vi "Actor Core.vi"(8 "error in":errorcluster, 11 "Select Report File Dialog in":refnum<class "Select Report File Dialog.lvclass">) -> (0 "error out":errorcluster, 3 "Actor out":refnum<class "Actor.lvclass">)   [LabVIEW 2014, in "Select Report File Dialog.lvlib" / "Select Report File Dialog.lvclass"]
doc: "(<B>Filename</B>: Actor Framework.lvlib:Actor.lvclass:Actor Core.vi)\n\nReceives messages to the actor, reacts to them, and initiates any error handling that may shut the actor down.\n\nDescendant classes may override this VI to append parallel tasks for the actor to complete while it handles messages. Overrides use the Call Parent Method node."
uses:
  Select Report File Dialog.lvclass
  <vilib>/ActorFramework/Actor/Actor.lvclass
  <vilib>/ActorFramework/Actor/Actor.lvclass/Actor.ctl
  <vilib>/ActorFramework/Message Enqueuer/Message Enqueuer.lvclass/Message Enqueuer.ctl
  Select Report File Dialog Messages/Write Select Report File Msg/Write Select Report File Msg.lvclass/Write Select Report File Msg.ctl
  <vilib>/ActorFramework/Message Enqueuer/Init from Existing Queue.vi
  <vilib>/ActorFramework/Message Enqueuer/Enqueue.vi
  <vilib>/ActorFramework/Message Priority Queue/Priority Enqueue.vi
  Viewable Actor/ViewableActor/ViewableActor.lvclass
  <vilib>/ActorFramework/Message Enqueuer/Message Enqueuer.lvclass
  Select Report File Dialog Messages/Write Select Report File Msg/Write Select Report File Msg.lvclass
  <vilib>/ActorFramework/Stop Msg/Stop Msg.lvclass
panel:
  in  "Select Report File":path
  in  "Stop Signal":bool
  in  "Stop":bool
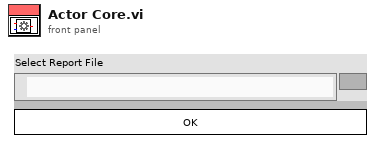
[diagram p1: front panel]
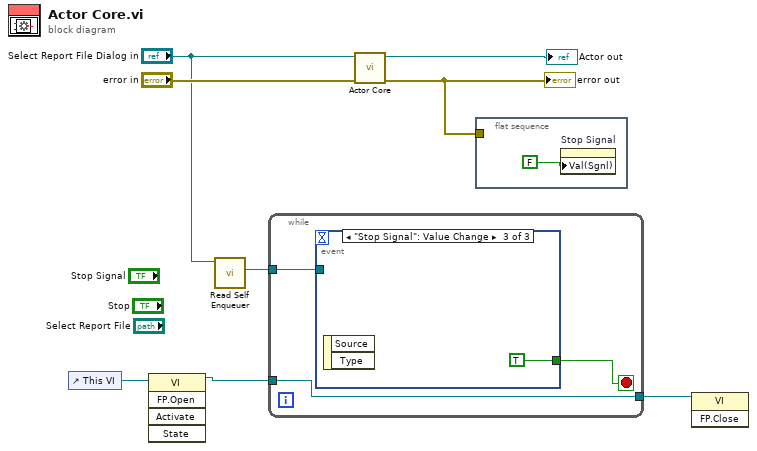
[diagram p0: block diagram]
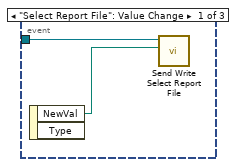
[diagram p2: hidden frame]
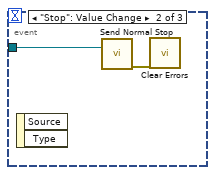
[diagram p3: hidden frame]
diagram:
  n1 = control-ref of="This VI"() -> (w3:refnum<vi>)
  n2 = invoke class="VI" method="FP.Open"(reference=w3) -> (reference out=w2:refnum<vi>)  [unwired: 4 in, 4 out]
  n3 = call <vilib>:"Read Self Enqueuer.vi"("Actor"="Select Report File Dialog in") -> ("Self Enqueuer"=w4:refnum<class "Message Enqueuer.lvclass">)  [unwired: 10 in]
  n4 = while {
    tunnel: w4 -> [w11]
    tunnel: w2 -> [w9]
    tunnel: [w9] -> w1
    stop <- w10 stop-if-true
    n5 = event shown="[2] \"Stop Signal\": Value Change" {
      selector: _ -> [_ _ _]
      dyn-events: _ -> [_ _ _]
      timeout: _ -> [_ _ _]
      tunnel: w11 -> [w12 w15 _]
      tunnel: [_ _ TRUE] -> w10
      event "Select Report File": Value Change {
        n6 = event-data() -> ("NewVal"=w13:path)  [unwired: 1 in, 1 out]
        n7 = call "Send Write Select Report File.vi"("Select Report File"=w13, "Message Enqueuer"=w12) -> ()  [unwired: 8 in, 2 out]
      }
      event "Stop": Value Change {
        n8 = event-data() -> ()  [unwired: 1 in, 2 out]
        n9 = call <vilib>:"Send Normal Stop.vi"("Message Enqueuer"=w15) -> ("error out"=w14:errorcluster)  [unwired: 10 in]
        n10 = call <vilib>:"Clear Errors.vi"("error in (no error)"=w14) -> ()  [unwired: 5 in, 2 out]
      }
      event "Stop Signal": Value Change {
        n11 = event-data() -> ()  [unwired: 1 in, 2 out]
      }
    }
  }
  n12 = call-parent "Actor Core.vi"("error in"="error in", "Actor in"="Select Report File Dialog in") -> ("error out"=w6:errorcluster, "Actor out"=→"Actor out":refnum<class "Actor.lvclass">)  [unwired: 8 in]
  "error out" <- w6
  n13 = flat-sequence {
    tunnel: w6 -> [_]
    frame #0 {
      n14 = property on="Stop Signal" class="Bool (strict)"("Val(Sgnl)"=FALSE ("Value (Signaling)")) -> ()  [unwired: 2 in, 2 out]
    }
  }
  n15 = invoke class="VI" method="FP.Close"(reference=w1) -> ()  [unwired: 2 in, 3 out]
